vi "Osci_saving Data in Excel.vi"() -> ()   [LabVIEW 2016]
doc: "This example shows how to use autosetup and acquire a waveform on a single channel."
uses:
  <instrlib>/Agilent 2000 3000 X-Series/Agilent 2000 3000 X-Series.lvlib
panel:
  in  "Probe Attenuation (10.0)":dbl=10.0
  out "Error_out":errorcluster
  in  "Error_in":errorcluster
  in  "stop":bool
  in  "Save":bool
  out "Waveform Data":waveform(dbl)(graph)
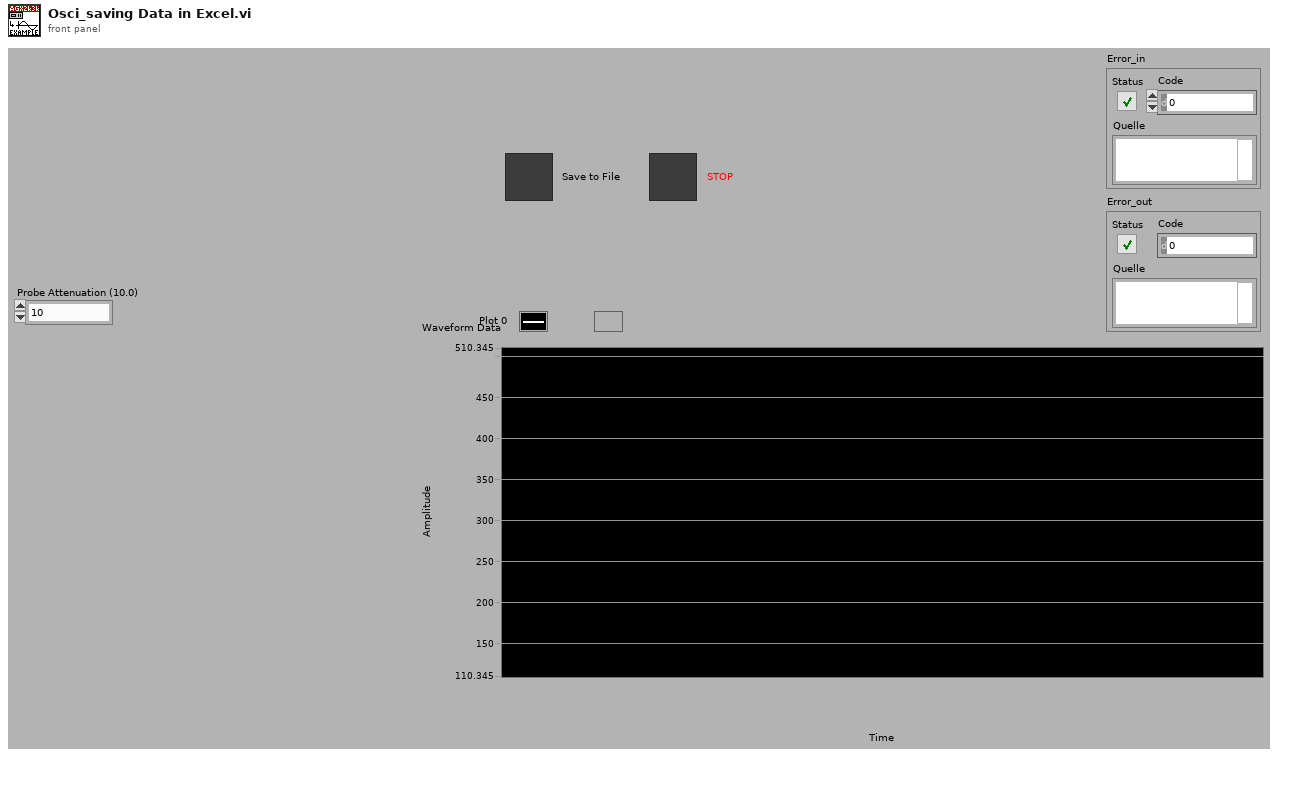
[diagram p1: front panel]
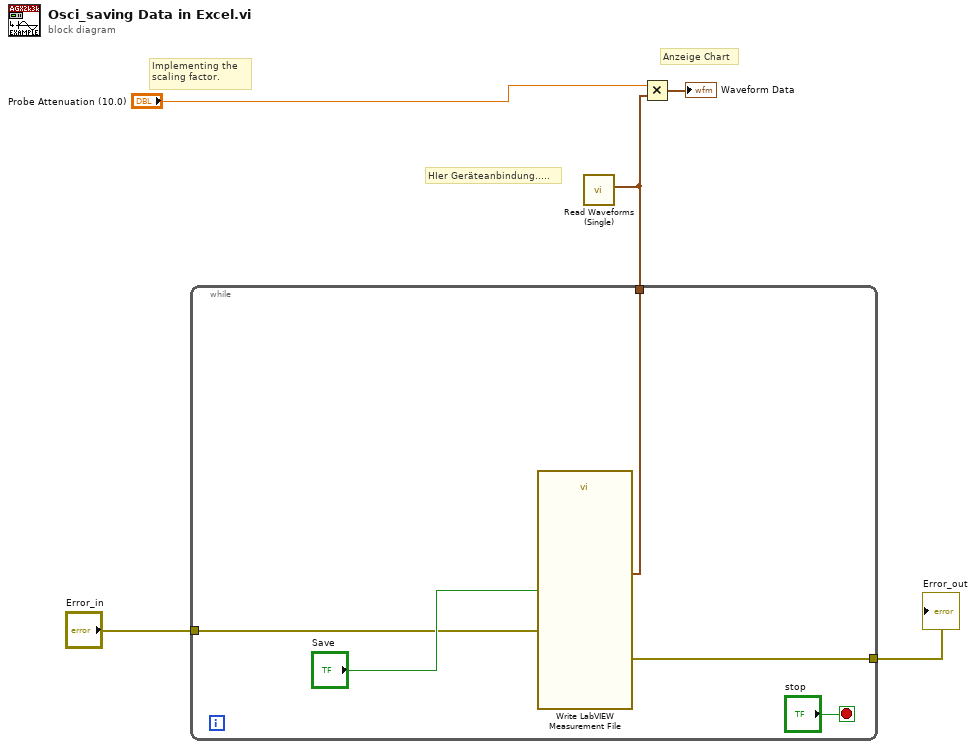
[diagram p0: block diagram]
diagram:
  # "Implementing the \nscaling factor."
  # "Anzeige Chart"
  # "HIer Geräteanbindung....."
  n1 = call <instrlib>:"Read Waveforms (Single).vi"() -> ("Waveform Data"=w4:waveform(dbl))  [unwired: 5 in, 6 out]
  n2 = while {
    tunnel: w4 -> [w8]
    tunnel: "Error_in" -> [w7]
    tunnel: [w6] -> w2
    stop <- "stop" stop-if-true
    n3 = call "Write LabVIEW Measurement File"("error in (no error)"=w7, "Enable"="Save", "Signals"=w8) -> ("error out"=w6:errorcluster)  [unwired: 6 in, 2 out]
  }
  "Error_out" <- w2
  n4 = Multiply(x="Probe Attenuation (10.0)", y=w4) -> (x*y=→"Waveform Data":waveform(dbl))
